vi "AttackerFSM.vi"(6 "Current State":dbl=1.0, 7 "IA State Input 2":T1, 8 "atacando contra?":bool=TRUE, 9 "balls":T4[](array[typedef])=[{"x"=-974.5169677734375, "y"=-3444.3310546875, "timestamp"=timestamp(2082759045.994995 s since 1904-01-01), "Vel_x"=0.0, "Vel_y"=0.0}], 10 "Field Size in":T5={"line_width"=10, "field_length"=9000, "field_width"=6000, "boundary_width"=250, "referee_width"=425, "goal_width"=700, "goal_depth"=180, "goal_wall_width"=20, "center_circle_radius"=500, "defense_radius"=500, "defense_stretch"=350, "free_kick_from_defense_dist"=700, "penalty_spot_from_field_line_dist"=450, "penalty_line_from_spot_dist"=350}, 11 "Robot in":T2={"id"=5, "function"=enum."Attacker", "x"=-983.1382446289062, "y"=-3000.010498046875, "orientation"=-1.5516623258590698, "v_tangent"=0.0, "v_normal"=0.0, "v_ang"=0.0, "kick_x"=0.0, "kick_z"=0.0, "dribble"=FALSE, "Timestamp"=timestamp(2082759045.994995 s since 1904-01-01), "dest_x"=0.0, "dest_y"=0.0, "dest_orientation"=0.0, "estimatives"={"est_v_tangent"=0.0, "est_v_normal"=0.0, "est_vx"=0.0, "est_vy"=0.0}}) -> (1 "Next State":dbl=1.0, 2 "Robot out":T2={"id"=5, "function"=enum."Attacker", "x"=-983.1382446289062, "y"=-3000.010498046875, "orientation"=-1.5516623258590698, "v_tangent"=0.0001540345015520423, "v_normal"=0.008599927144915481, "v_ang"=0.002668461263266586, "kick_x"=0.0, "kick_z"=0.0, "dribble"=FALSE, "Timestamp"=timestamp(2082759045.994995 s since 1904-01-01), "dest_x"=0.0, "dest_y"=0.0, "dest_orientation"=0.0, "estimatives"={"est_v_tangent"=0.0, "est_v_normal"=0.0, "est_vx"=0.0, "est_vy"=0.0}})   [LabVIEW 2016]
uses:
  Core/AI Robot.ctl
  Functions Enum.ctl
  Core/Field Size.ctl
  Core/AI Ball.ctl
  Core/AI Input.ctl
  Core/AI Judge.ctl
  Command Enum.ctl
  <vilib>/Analysis/coordinate.llb/2D Cartesian Coordinate Rotation (Scalar).vi
  <vilib>/Analysis/NI_AALPro.lvlib
panel:
  in  "attacker farback":dbl=1500.0 format="%#_13g"
  out "Elapsed Time (s) 2":dbl caption="Elapsed Time (s)"
  in  "reckon timer":dbl=1.0 caption="Time Target (s)"
  in  "distance between ball and robot":dbl=275.0 format="%#_13g"
  out "Waveform Chart":dbl(graph)
  out "Elapsed Time (s)":dbl
  in  "Time Target \nto transition":dbl=1.0 caption="Time Target (s)"
  in  "Dist a frente da bola":dbl format="%#_13g"
  in  "Longe":dbl=300.0 format="%#_13g"
  in  "raio da circunferencia":dbl=175.0 format="%#_13g"
  in  "Cone de rotação":dbl=1.1 format="%#_13g"
  in  "Cone de chute":dbl=0.09 format="%#_13g"
  in  "Perto":dbl=300.0 format="%#_13g"
  in  "min dist to kick":dbl=165.0 format="%#_13g"
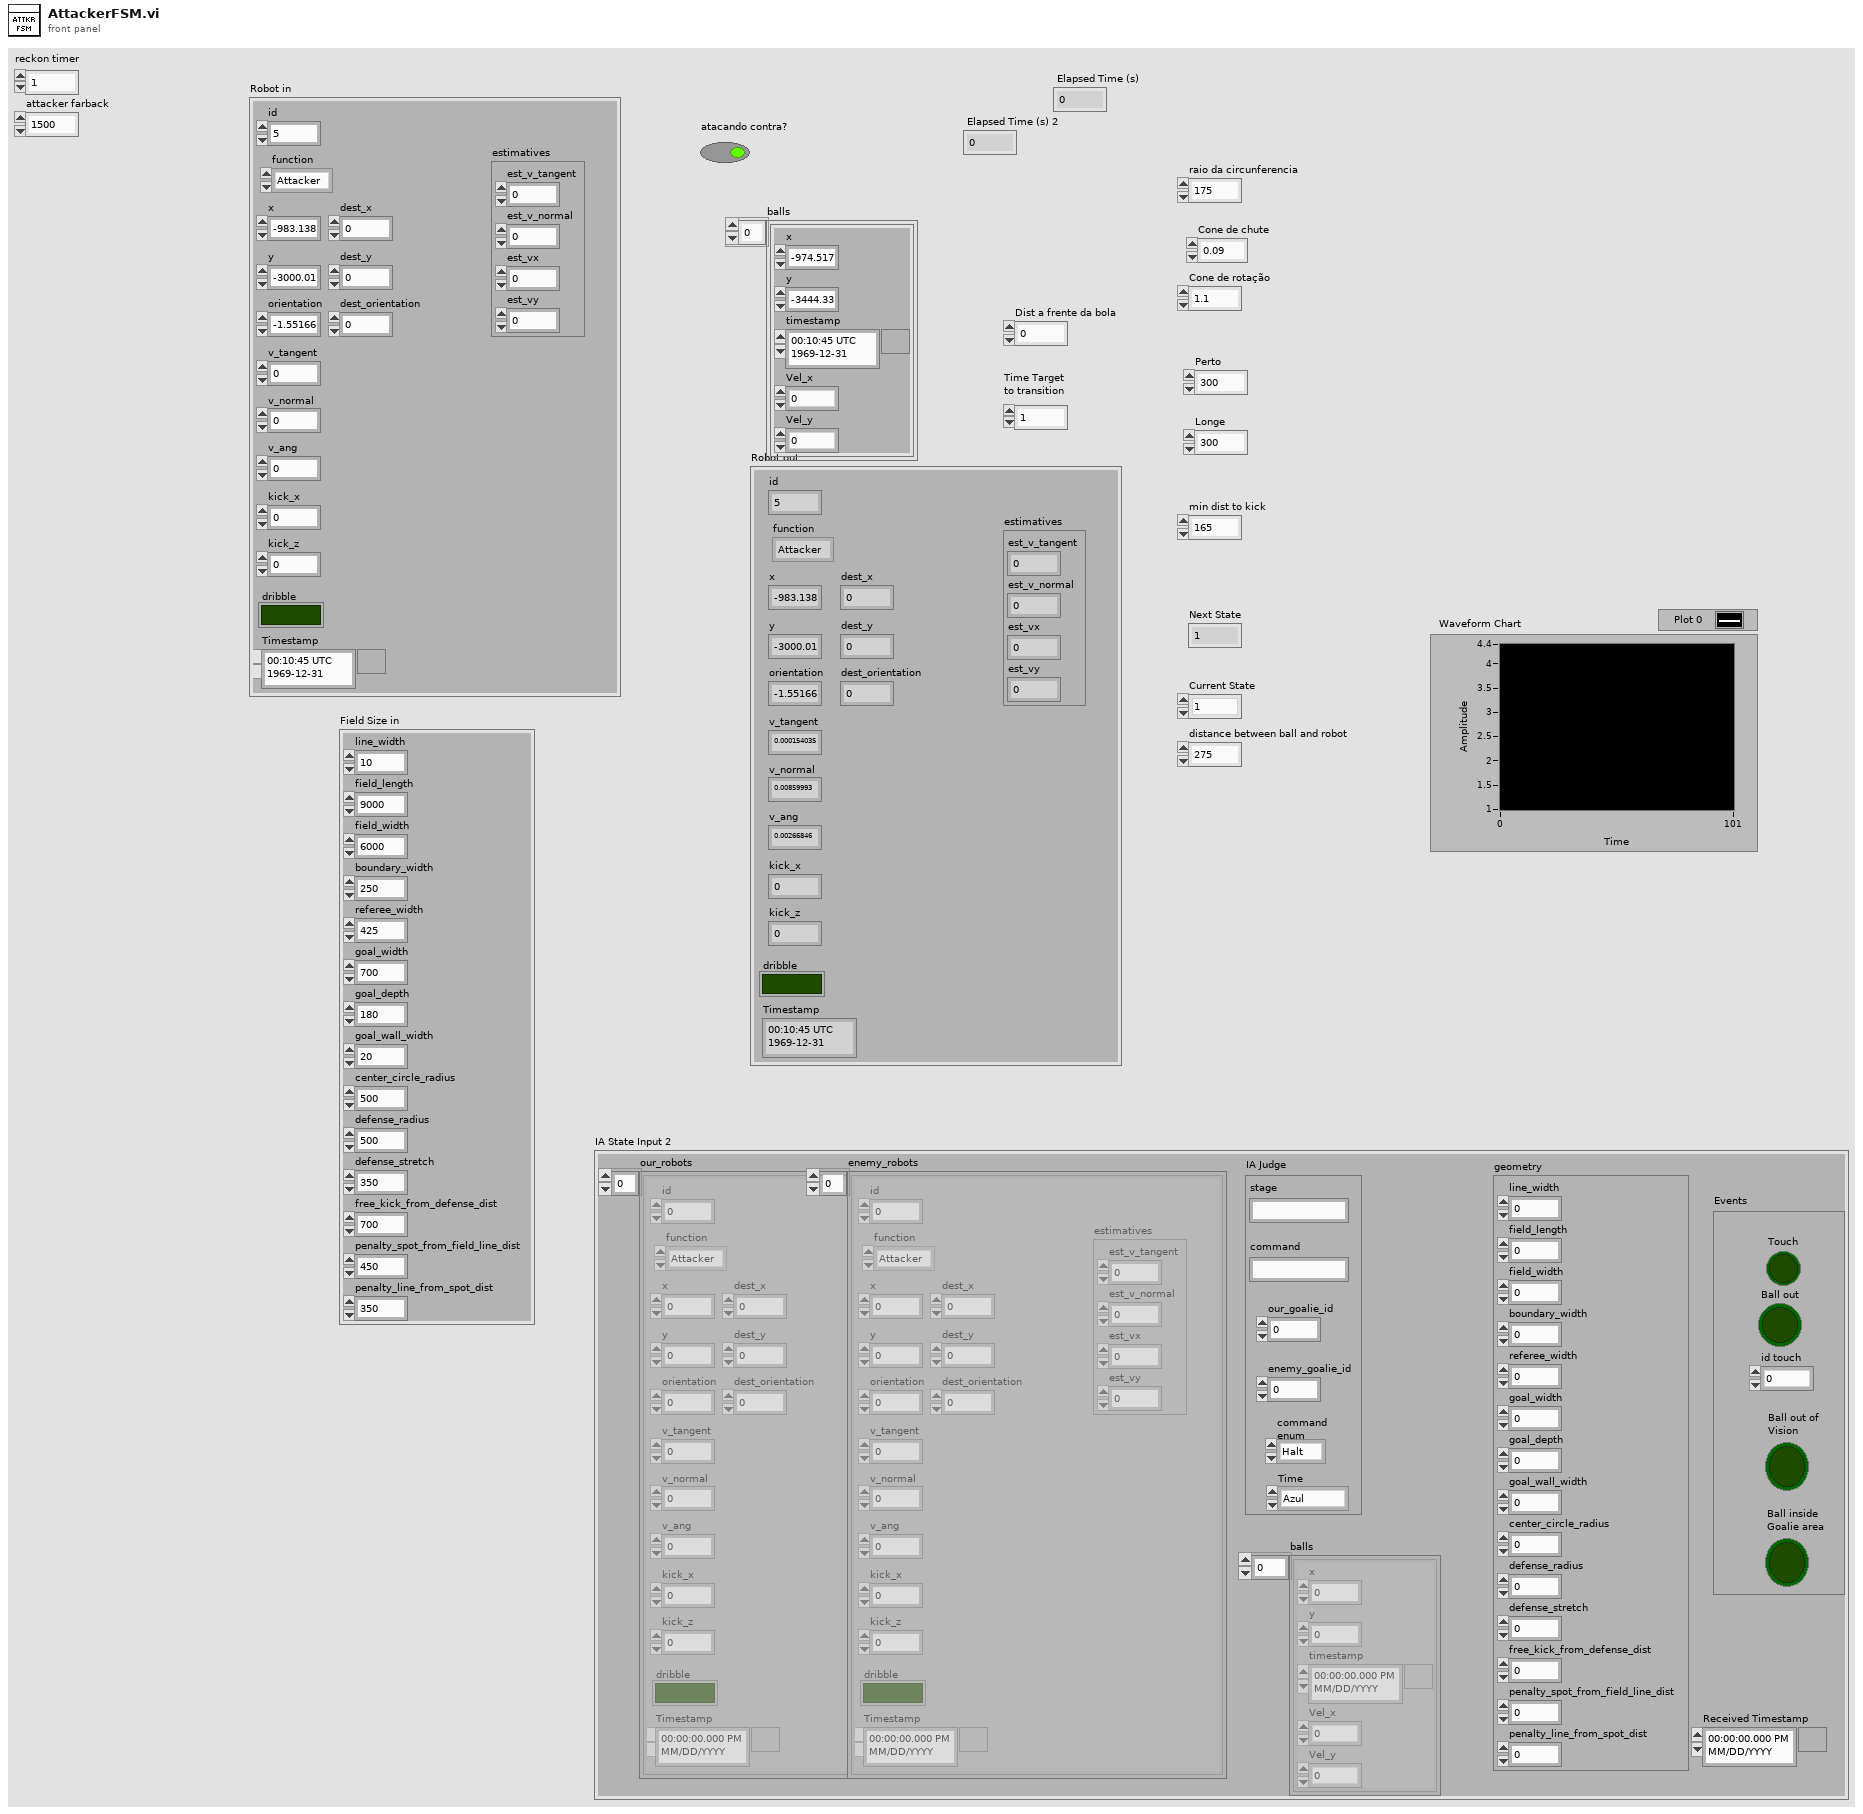
[diagram p1: front panel]
types:
  T1 = typedef "AI Input.ctl" = cluster{"our_robots":T2[], "enemy_robots":T2[], "balls":T4[], "geometry":T5, "IA Judge":T6, "Received Timestamp":timestamp, "Events":cluster{"Touch":bool, "Ball out":bool, "id touch":dbl, "Ball out of \nVision":bool, "Ball inside \nGoalie area":bool}}
  T2 = typedef "AI Robot.ctl" = cluster{"id":u32, "function":T3, "x":dbl, "y":dbl, "orientation":dbl, "v_tangent":dbl, "v_normal":dbl, "v_ang":dbl, "kick_x":dbl, "kick_z":dbl, "dribble":bool, "Timestamp":timestamp, "dest_x":dbl, "dest_y":dbl, "dest_orientation":dbl, "estimatives":cluster{"est_v_tangent":dbl, "est_v_normal":dbl, "est_vx":dbl, "est_vy":dbl}}
  T3 = typedef "Functions Enum.ctl" = enum16{"Attacker", "Goalie", "Defender", "Striker", "Goto 0", "Dummy", "ZigZag"}
  T4 = typedef "AI Ball.ctl" = cluster{"x":dbl, "y":dbl, "timestamp":timestamp, "Vel_x":dbl, "Vel_y":dbl}
  T5 = typedef "Field Size.ctl" = cluster{"line_width":u32, "field_length":u32, "field_width":u32, "boundary_width":u32, "referee_width":u32, "goal_width":u32, "goal_depth":u32, "goal_wall_width":u32, "center_circle_radius":u32, "defense_radius":u32, "defense_stretch":u32, "free_kick_from_defense_dist":u32, "penalty_spot_from_field_line_dist":u32, "penalty_line_from_spot_dist":u32}
  T6 = typedef "AI Judge.ctl" = cluster{"stage":string, "command":string, "our_goalie_id":dbl, "enemy_goalie_id":dbl, "command\nenum":T7, "Time":enum16{"Azul", "Amarelo"}}
  T7 = typedef "Command Enum.ctl" = enum16{"Halt", "Stop", "Force Start", "PKA Normal Start", "Prepare Kickoff Ally", "PKE Normal Start", "Prepare Kickoff Enemy", "Prepare Penalty Ally", "PPA Normal Start", "Prepare Penalty Enemy", "PPE Normal Start", "Direct Free Enemy", "Direct Free Ally", "Indirect Free Enemy", "Indirect Free Ally", "Timeout Enemy", "Timeout Ally", "Goal Enemy", "Goal Ally", "Ball Placement Enemy", "Ball Placement Ally", "None"}
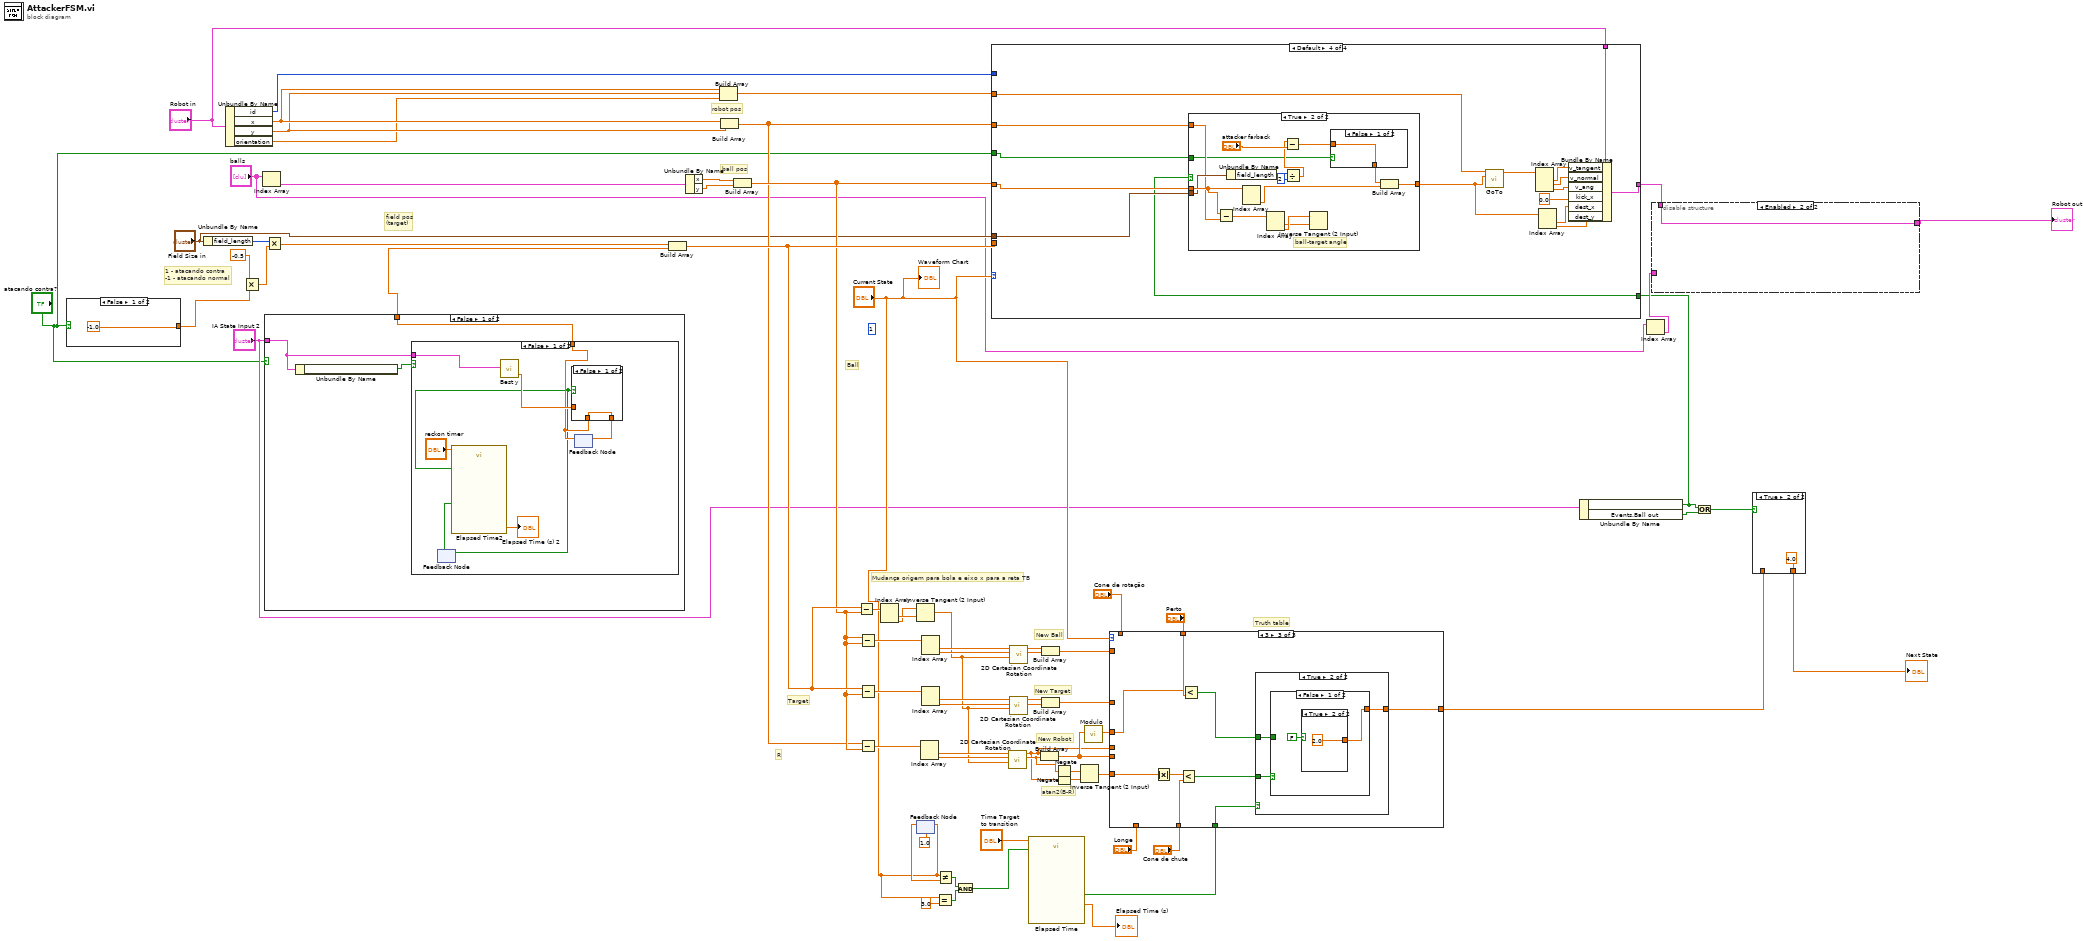
[diagram p0: block diagram]
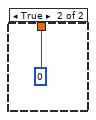
[diagram p3: hidden frame]
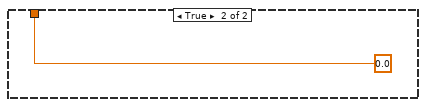
[diagram p4: hidden frame]
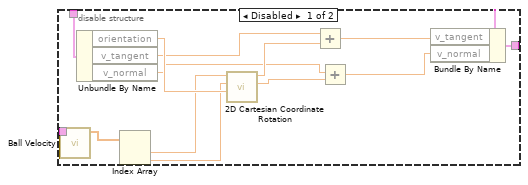
[diagram p5: hidden frame]
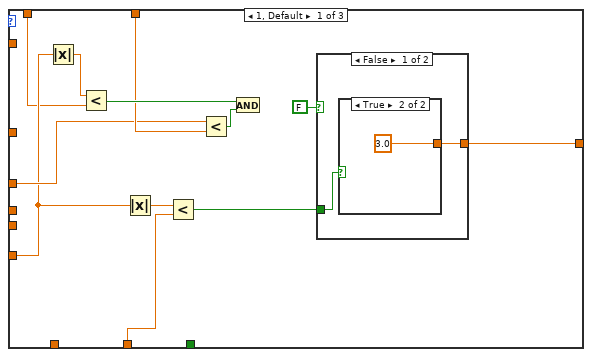
[diagram p6: hidden frame]
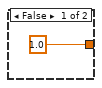
[diagram p7: hidden frame]
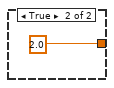
[diagram p8: hidden frame]
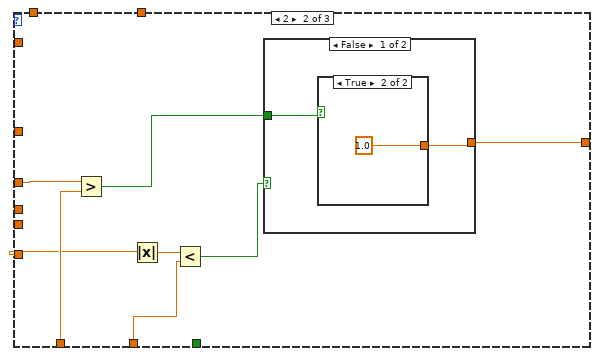
[diagram p9: hidden frame]
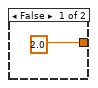
[diagram p10: hidden frame]
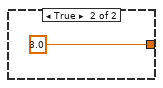
[diagram p11: hidden frame]
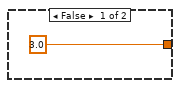
[diagram p12: hidden frame]
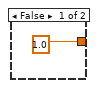
[diagram p13: hidden frame]
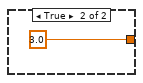
[diagram p14: hidden frame]
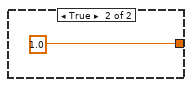
[diagram p16: hidden frame]
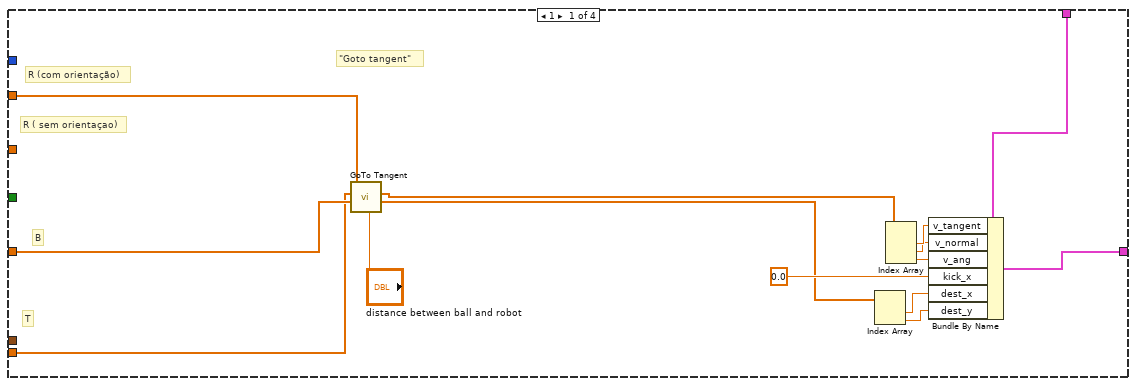
[diagram p17: hidden frame]
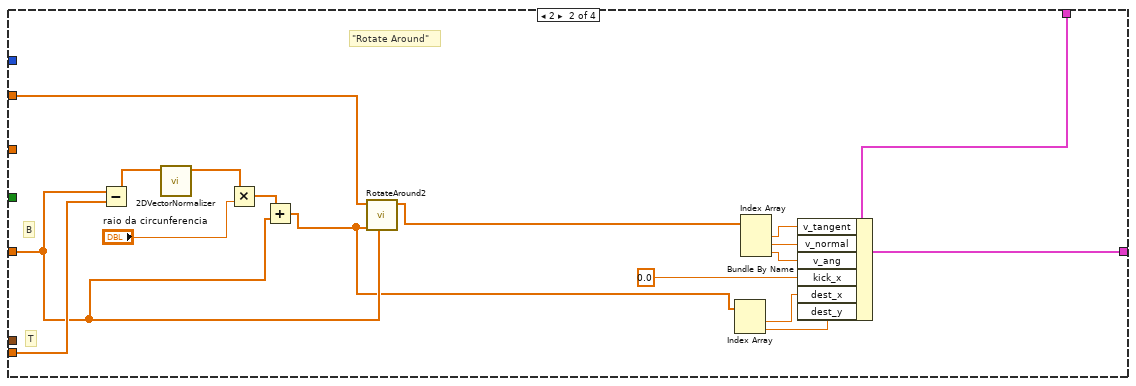
[diagram p18: hidden frame]
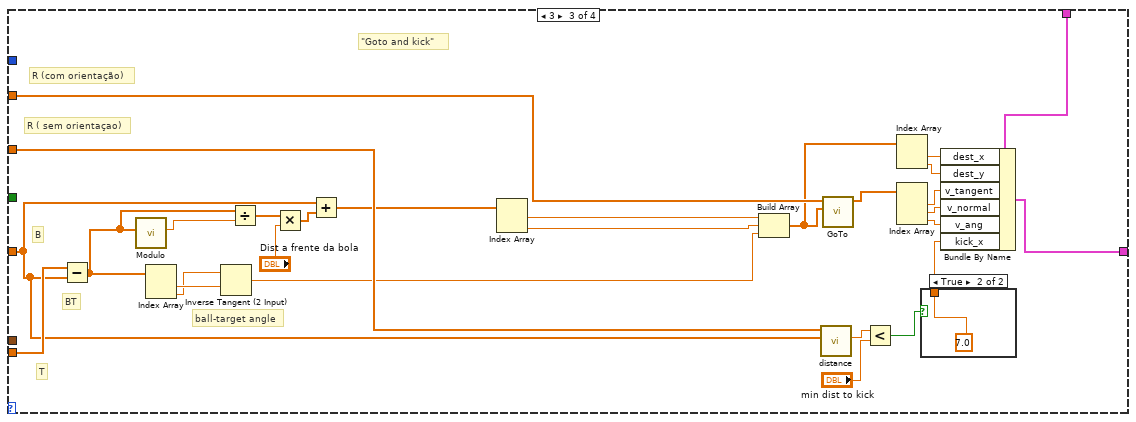
[diagram p19: hidden frame]
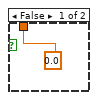
[diagram p20: hidden frame]
diagram:
  (unwired) 1
  # "atan2(B-R)"
  # "New Robot"
  # "New Target"
  # "New Ball"
  # "R"
  # "Ball"
  # "Target"
  # "Mudança origem para bola e eixo x para a reta TB"
  # "1 - atacando contra\n-1 - atacando normal"
  # "Truth table"
  # "robot pos"
  # "field pos\n(target)"
  # "ball pos"
  n1 = case shown="False" "atacando contra?" {
    tunnel: [-1.0 ("attck contra? 2") 1.0] -> w29
    frame False {
    }
    frame True {
    }
  }
  n2 = Unbundle By Name("Field Size in") -> ("field_length"=w69:u32)
  n3 = Unbundle By Name("Robot in") -> ("id"=w23:u32, "x"=w65:dbl, "y"=w64:dbl, "orientation"=w61:dbl)
  n4 = Multiply(x=-0.5, y=w29) -> (x*y=w59:dbl)
  n5 = Index Array(array="balls") -> (element=w70:T4)  [unwired: 1 in]
  n6 = case shown="False" "atacando contra?" {
    tunnel: "IA State Input 2" -> [w73 _]
    tunnel: [w74 0.0 ("element")] -> w6
    frame False {
      n7 = Unbundle By Name(w73) -> ("Events.Ball inside \nGoalie area"=w75:bool)
      n8 = case shown="False" w75 {
        tunnel: [w80 0] -> w74
        tunnel: w73 -> [w83 _]
        frame False {
          n9 = feedback #1() -> (w76:bool)  [unwired: 1 in]
          n10 = call "Elapsed Time2"("Time Target (s)"="reckon timer", "Auto Reset"=w76) -> ("Elapsed Time (s)"=→"Elapsed Time (s) 2":dbl, "Time has Elapsed"=w77:bool)  [unwired: 10 in, 6 out]
          n11 = feedback-in #1(w77) -> ()
          n12 = call "Best y.vi"("IA State"=w83) -> ("Best y"=w82:dbl)  [unwired: 5 in, 5 out]
          n13 = feedback #2() -> (w80:dbl)  [unwired: 1 in]
          n14 = case shown="False" w76 {
            tunnel: w82 -> [_ w85]
            tunnel: [w84 w85] -> w81
            tunnel: w80 -> [w84 _]
            frame False {
            }
            frame True {
            }
          }
          n15 = feedback-in #2(w81) -> ()
        }
        frame True {
        }
      }
    }
    frame True {
    }
  }
  n16 = Multiply(x=w69, y=w59) -> (x*y=w68:dbl)
  n17 = Build Array(w68, w6) -> (w41:dbl[])
  n18 = Unbundle By Name(w70) -> ("x"=w67:dbl, "y"=w66:dbl)
  n19 = Build Array(w65, w64, w61) -> (w62:dbl[])
  n20 = Build Array(w65, w64) -> (w39:dbl[])
  n21 = Build Array(w67, w66) -> (w40:dbl[])
  n22 = Subtract(x=w41, y=w40) -> (x-y=w49:dbl[])
  n23 = Subtract(x=w40, y=w40) -> (x-y=w56:dbl[])
  n24 = Subtract(x=w41, y=w40) -> (x-y=w53:dbl[])
  n25 = Subtract(x=w39, y=w40) -> (x-y=w50:dbl[])
  n26 = Index Array(array=w49) -> (element #1=w48:dbl, element #2=w47:dbl)  [unwired: 2 in]
  n27 = Inverse Tangent (2 Input)(1:w48, 2:w47) -> (0:w42:dbl)
  n28 = feedback-in #3("Current State") -> ()
  n29 = feedback #3(1.0 ("Current State")) -> (w15:dbl)
  n30 = Index Array(array=w50) -> (element #1=w52:dbl, element #2=w51:dbl)  [unwired: 2 in]
  n31 = Index Array(array=w53) -> (element #1=w55:dbl, element #2=w54:dbl)  [unwired: 2 in]
  n32 = Index Array(array=w56) -> (element #1=w58:dbl, element #2=w57:dbl)  [unwired: 2 in]
  n33 = Equal?(x="Current State", y=3.0) -> (x = y?=w19:bool)
  n34 = Not Equal?(x="Current State", y=w15) -> (x != y?=w18:bool)
  n35 = And(x=w18, y=w19) -> (x .and. y?=w13:bool)
  n36 = call-poly <vilib>:"2D Cartesian Coordinate Rotation.vi"("theta"=w42, "y"=w51, "x"=w52) -> ("y out"=w26:dbl, "x out"=w25:dbl)  [unwired: 6 in, 1 out]
  n37 = call-poly <vilib>:"2D Cartesian Coordinate Rotation.vi"("theta"=w42, "y"=w54, "x"=w55) -> ("y out"=w45:dbl, "x out"=w46:dbl)  [unwired: 6 in, 1 out]
  n38 = call-poly <vilib>:"2D Cartesian Coordinate Rotation.vi"("theta"=w42, "y"=w57, "x"=w58) -> ("y out"=w43:dbl, "x out"=w44:dbl)  [unwired: 6 in, 1 out]
  n39 = call "Elapsed Time"("Time Target (s)"="Time Target \nto transition", "Reset"=w13) -> ("Elapsed Time (s)"=→"Elapsed Time (s)":dbl, "Time has Elapsed"=w21:bool)  [unwired: 10 in, 6 out]
  n40 = Build Array(w25, w26) -> (w34:dbl[])
  n41 = Build Array(w46, w45) -> (w35:dbl[])
  n42 = Build Array(w44, w43) -> (w36:dbl[])
  n43 = Negate(x=w26) -> (-x=w28:dbl)
  n44 = Negate(x=w25) -> (-x=w27:dbl)
  n45 = Inverse Tangent (2 Input)(1:w27, 2:w28) -> (0:w32:dbl)
  n46 = call "Modulo.vi"("2D vector"=w34) -> ("Modulo"=w33:dbl)  [unwired: 10 in]
  n47 = case shown="3" "Current State" {
    tunnel: "Longe" -> [_ w111 _]
    tunnel: "Cone de chute" -> [w93 w106 w121]
    tunnel: w36 -> [_ _ _]
    tunnel: w35 -> [_ _ _]
    tunnel: w34 -> [_ _ _]
    tunnel: w33 -> [w96 w112 w124]
    tunnel: w32 -> [w91 w107 w122]
    tunnel: [w95 w110 w126] -> w31
    tunnel: "Perto" -> [w97 _ w125]
    tunnel: w25 -> [_ _ _]
    tunnel: w21 -> [_ _ w118]
    tunnel: "Cone de rotação" -> [w89 _ _]
    frame 1, Default {
      n48 = Absolute Value(x=w91) -> (abs(x)=w90:dbl)
      n49 = Less?(x=w90, y=w89) -> (x < y?=w99:bool)
      n50 = Absolute Value(x=w91) -> (abs(x)=w94:dbl)
      n51 = Less?(x=w94, y=w93) -> (x < y?=w92:bool)
      n52 = Less?(x=w96, y=w97) -> (x < y?=w98:bool)
      n53 = And(x=w99, y=w98) -> ()  [unwired: 1 out]
      n54 = case shown="False" FALSE {
        tunnel: [w101 2.0] -> w95
        tunnel: w92 -> [w100 _]
        frame False {
          n55 = case shown="True" w100 {
            tunnel: [1.0 3.0] -> w101
            frame False {
            }
            frame True {
            }
          }
        }
        frame True {
        }
      }
    }
    frame 2 {
      n56 = Greater?(x=w112, y=w111) -> (0:w109:bool)
      n57 = Absolute Value(x=w107) -> (abs(x)=w108:dbl)
      n58 = Less?(x=w108, y=w106) -> (x < y?=w105:bool)
      n59 = case shown="False" w105 {
        tunnel: [w113 3.0] -> w110
        tunnel: w109 -> [w114 _]
        frame False {
          n60 = case shown="True" w114 {
            tunnel: [2.0 1.0] -> w113
            frame False {
            }
            frame True {
            }
          }
        }
        frame True {
        }
      }
    }
    frame 3 {
      n61 = Absolute Value(x=w122) -> (abs(x)=w123:dbl)
      n62 = Less?(x=w123, y=w121) -> (x < y?=w120:bool)
      n63 = Less?(x=w124, y=w125) -> (x < y?=w119:bool)
      n64 = case shown="True" w118 {
        tunnel: [3.0 w130] -> w126
        tunnel: w120 -> [_ w129]
        tunnel: w119 -> [_ w128]
        frame False {
        }
        frame True {
          n65 = case shown="False" w129 {
            tunnel: [w132 3.0] -> w130
            tunnel: w128 -> [_ _]
            frame False {
              n66 = case shown="True" FALSE {
                tunnel: [1.0 2.0] -> w132
                frame False {
                }
                frame True {
                }
              }
            }
            frame True {
            }
          }
        }
      }
    }
  }
  n67 = Unbundle By Name("IA State Input 2") -> ("Events.Ball inside \nGoalie area"=w2:bool, "Events.Ball out"=w4:bool)
  n68 = case shown="Default" "Current State" {
    tunnel: [w149 w166 w194 w212] -> w10
    tunnel: "Robot in" -> [w148 w154 w193 w211]
    tunnel: w62 -> [w146 w165 w180 w203]
    tunnel: w39 -> [_ _ w188 w205]
    tunnel: w40 -> [w142 w153 w170 w206]
    tunnel: w41 -> [w141 w159 w185 _]
    tunnel: "Field Size in" -> [_ _ _ w204]
    tunnel: w23 -> [_ _ _ _]
    tunnel: w2 -> [_ _ _ w198]
    tunnel: "atacando contra?" -> [_ _ _ w197]
    frame 1 {
      # "\"Goto tangent\""
      # "B"
      # "T"
      # "R ( sem orientaçao)"
      # "R (com orientação)"
      n69 = call "GoTo Tangent.vi"("distance between ball and robot"="distance between ball and robot", "Ball"=w142, "Target"=w141, "R"=w146) -> ("Destination"=w138:dbl[], "Output\nVelocity"=w140:dbl[])  [unwired: 6 in]
      n70 = Index Array(array=w138) -> (element #1=w137:dbl, element #2=w136:dbl)  [unwired: 2 in]
      n71 = Index Array(array=w140) -> (element #1=w145:dbl, element #2=w144:dbl, element #3=w143:dbl)  [unwired: 3 in]
      n72 = Bundle By Name(cluster=w148, "v_tangent"=w145, "v_normal"=w144, "v_ang"=w143, "kick_x"=0.0, "dest_x"=w137, "dest_y"=w136) -> (w149:T2)
    }
    frame 2 {
      # "T"
      # "B"
      # "\"Rotate Around\""
      n73 = Subtract(x=w153, y=w159) -> (x-y=w158:dbl[])
      n74 = call "2DVectorNormalizer.vi"("2D vector"=w158) -> ("2D vector 2"=w157:dbl[])  [unwired: 10 in]
      n75 = Multiply(x=w157, y="raio da circunferencia") -> (x*y=w155:dbl[])
      n76 = Add(x=w155, y=w153) -> (x+y=w152:dbl[])
      n77 = call "RotateAround2.vi"("Centre"=w153, "Target"=w152, "Position"=w165) -> ("Output\nVelocity"=w160:dbl[])  [unwired: 8 in]
      n78 = Index Array(array=w152) -> (element #1=w151:dbl, element #2=w150:dbl)  [unwired: 2 in]
      n79 = Index Array(array=w160) -> (element #1=w163:dbl, element #2=w162:dbl, element #3=w161:dbl)  [unwired: 3 in]
      n80 = Bundle By Name(cluster=w154, "v_tangent"=w163, "v_normal"=w162, "v_ang"=w161, "kick_x"=0.0, "dest_x"=w151, "dest_y"=w150) -> (w166:T2)
    }
    frame 3 {
      # "BT"
      # "ball-target angle"
      # "B"
      # "T"
      # "R ( sem orientaçao)"
      # "R (com orientação)"
      # "\"Goto and kick\""
      n81 = Subtract(x=w185, y=w170) -> (x-y=w171:dbl[])
      n82 = call "Modulo.vi"("2D vector"=w171) -> ("Modulo"=w172:dbl)  [unwired: 10 in]
      n83 = Index Array(array=w171) -> (element #1=w187:dbl, element #2=w186:dbl)  [unwired: 2 in]
      n84 = Inverse Tangent (2 Input)(1:w187, 2:w186) -> (0:w184:dbl)
      n85 = Divide(x=w171, y=w172) -> (x/y=w173:dbl[])
      n86 = Multiply(x=w173, y="Dist a frente da bola") -> (x*y=w176:dbl[])
      n87 = Add(x=w170, y=w176) -> (x+y=w174:dbl[])
      n88 = Index Array(array=w174) -> (element #1=w183:dbl, element #2=w182:dbl)  [unwired: 2 in]
      n89 = Build Array(w183, w182, w184) -> (w168:dbl[])
      n90 = call "distance.vi"("target pos"=w170, "obj pos"=w188) -> ("sqrt(x)"=w192:dbl)  [unwired: 9 in]
      n91 = call "GoTo.vi"("Target"=w168, "Position"=w180) -> ("Output\nVelocity"=w181:dbl[])  [unwired: 8 in, 1 out]
      n92 = Less?(x=w192, y="min dist to kick") -> (x < y?=w190:bool)
      n93 = Index Array(array=w168) -> (element #1=w169:dbl, element #2=w167:dbl)  [unwired: 2 in]
      n94 = Index Array(array=w181) -> (element #1=w179:dbl, element #2=w178:dbl, element #3=w177:dbl)  [unwired: 3 in]
      n95 = case shown="True" w190 {
        tunnel: [0.0 7.0] -> w191
        frame False {
        }
        frame True {
        }
      }
      n96 = Bundle By Name(cluster=w193, "dest_x"=w169, "dest_y"=w167, "v_tangent"=w179, "v_normal"=w178, "v_ang"=w177, "kick_x"=w191) -> (w194:T2)
    }
    frame Default {
      n97 = case shown="True" w198 {
        tunnel: w206 -> [w216 w225]
        tunnel: w205 -> [w215 w221]
        tunnel: w204 -> [w214 w224]
        tunnel: [w213 w230] -> w201
        tunnel: w197 -> [_ w217]
        frame False {
          n98 = call "PosBolaFora.vi"("Field Size in"=w214, "Position da bola"=w216, "Position do robot"=w215) -> ("Target"=w213:dbl[])  [unwired: 8 in]
        }
        frame True {
          # "ball-target angle"
          n99 = Subtract(x=w225, y=w221) -> (x-y=w228:dbl[])
          n100 = Unbundle By Name(w224) -> ("field_length"=w220:u32)
          n101 = Index Array(array=w225) -> (element #2=w231:dbl)  [unwired: 2 in, 1 out]
          n102 = Index Array(array=w228) -> (element #1=w226:dbl, element #2=w227:dbl)  [unwired: 2 in]
          n103 = Divide(x=w220, y=u32 2) -> (x/y=w218:dbl)
          n104 = Subtract(x=w218, y="attacker farback") -> (x-y=w223:dbl)
          n105 = Inverse Tangent (2 Input)(1:w226, 2:w227) -> ()  [unwired: 1 out]
          n106 = case shown="False" w217 {
            tunnel: w223 -> [w232 w235]
            tunnel: [w232 w234] -> w229
            frame False {
            }
            frame True {
              n107 = Multiply(x=w235, y=-1.0) -> (x*y=w234:dbl)
            }
          }
          n108 = Build Array(w229, w231) -> (w230:dbl[])
        }
      }
      n109 = call "GoTo.vi"("Target"=w201, "Position"=w203) -> ("Output\nVelocity"=w202:dbl[])  [unwired: 8 in, 1 out]
      n110 = Index Array(array=w202) -> (element #1=w209:dbl, element #2=w208:dbl, element #3=w207:dbl)  [unwired: 3 in]
      n111 = Index Array(array=w201) -> (element #1=w200:dbl, element #2=w199:dbl)  [unwired: 2 in]
      n112 = Bundle By Name(cluster=w211, "v_tangent"=w209, "v_normal"=w208, "v_ang"=w207, "kick_x"=0.0, "dest_x"=w200, "dest_y"=w199) -> (w212:T2)
    }
  }
  n113 = Index Array(array="balls") -> (element=w8:T4)  [unwired: 1 in]
  n114 = disable-structure shown="Enabled" {
    disable-tunnel: w10 -> [w240 w249]
    disable-tunnel: [w237 w249] -> w9
    disable-tunnel: w8 -> [w236 _]
    frame Disabled {
      n115 = call "Ball Velocity.vi"("Ball"=w236) -> ("Velocity"=w247:dbl[])  [unwired: 10 in]
      n116 = Unbundle By Name(w240) -> ("orientation"=w248:dbl, "v_tangent"=w243:dbl, "v_normal"=w241:dbl)
      n117 = Index Array(array=w247) -> (element #1=w245:dbl, element #2=w246:dbl)  [unwired: 2 in]
      n118 = call-poly <vilib>:"2D Cartesian Coordinate Rotation.vi"("theta"=w248, "y"=w246, "x"=w245) -> ("y out"=w242:dbl, "x out"=w244:dbl)  [unwired: 6 in, 1 out]
      n119 = Add(x=w243, y=w244) -> (x+y=w239:dbl)
      n120 = Add(x=w241, y=w242) -> (x+y=w238:dbl)
      n121 = Bundle By Name(cluster=w240, "v_tangent"=w239, "v_normal"=w238) -> (w237:T2)
    }
    frame Enabled {
    }
  }
  "Robot out" <- w9
  n122 = Or(x=w2, y=w4) -> (x .or. y?=w3:bool)
  n123 = case shown="True" w3 {
    tunnel: [w250 4.0] -> w16
    tunnel: w31 -> [w250 _]
    frame False {
    }
    frame True {
    }
  }
  "Next State" <- w16
  "Waveform Chart" <- "Current State"
